vi "ActiveObject_QueueQueue_Process.vi"(0 "reference in":refnum<class>, 5 "error in (no error)":errorcluster) -> (14 "reference out":refnum<class>, 19 "error out":errorcluster)   [LabVIEW 2010]
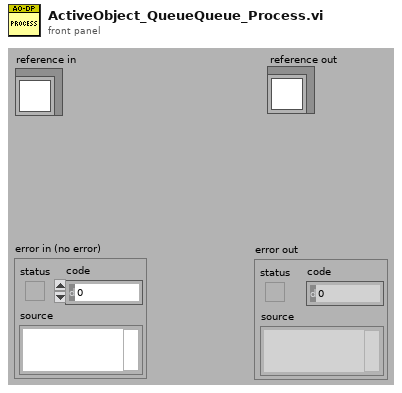
[diagram p1: front panel]
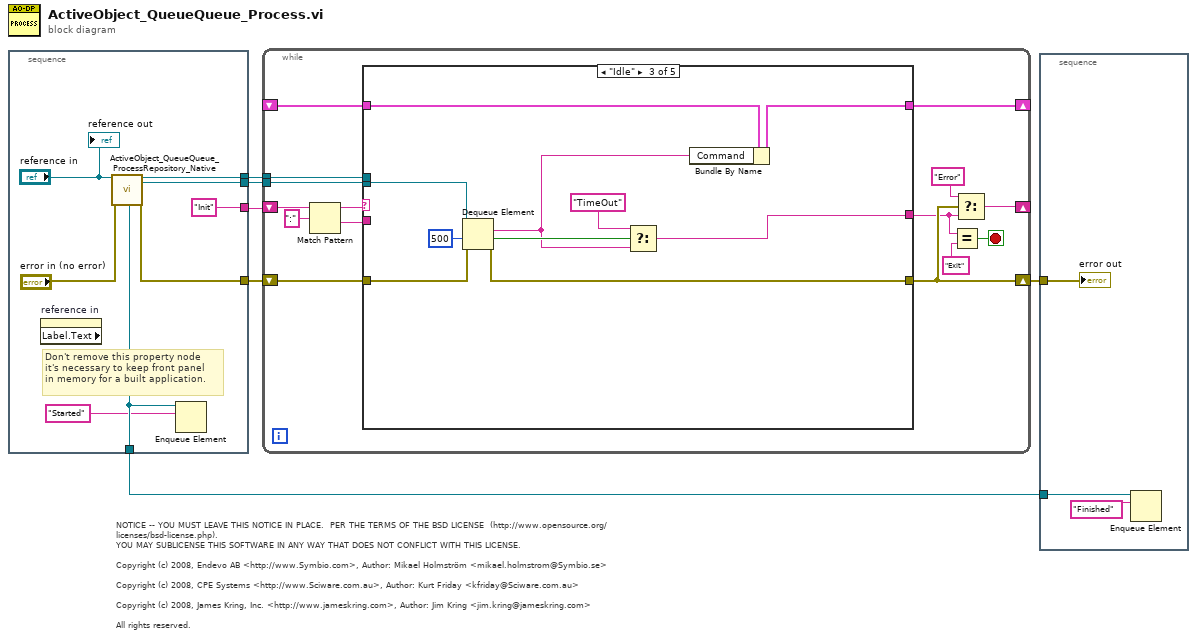
[diagram p0: block diagram]
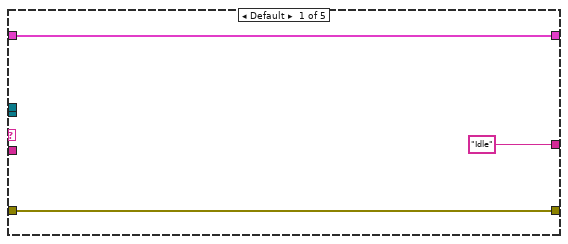
[diagram p2: hidden frame]
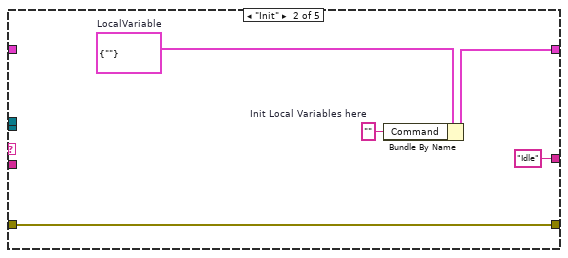
[diagram p3: hidden frame]
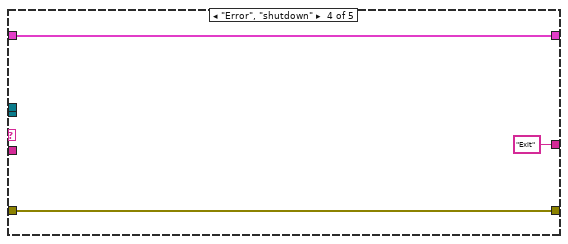
[diagram p4: hidden frame]
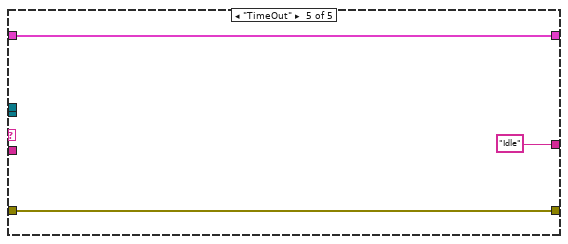
[diagram p5: hidden frame]
diagram:
  # "NOTICE -- YOU MUST LEAVE THIS NOTICE IN PLACE.  PER THE TERMS OF THE BSD LICENSE  (http://www.opensource.org/licenses/bsd-license.php).\nYOU MAY SUBLICENSE THIS SOFTWARE IN ANY WAY THAT DOES NOT CONFLICT WITH THIS LICENSE.\n\nCopyright (c) 2008, Endevo AB <http://www.Symbio.com>, Author: Mikael Holmström <mikael.holmstrom@Symbio.se>\n\nCopyright (c) 2008, CPE Systems <http://www.Sciware.com.au>, Author: Kurt Friday <kfriday@Sciware.com.au>\n\nCopyright (c) 2008, James Kring, Inc. <http://www.jameskring.com>, Author: Jim Kring <jim.kring@jameskring.com>\n\nAll rights reserved."
  n1 = stacked-sequence {
    tunnel: [w11] -> w6
    tunnel: [w14] -> w4
    tunnel: [w10] -> w3
    tunnel: [w8] -> w2
    tunnel: ["Init"] -> w1
    frame #0 {
      # "Don't remove this property node\nit's necessary to keep front panel\nin memory for a built application."
      n2 = property on="reference in" class="LVClassControl (strict)" props=["Label", "Text"]() -> ()  [unwired: 2 in, 3 out]
      n3 = call "ActiveObject_QueueQueue_ProcessRepository_Native.vi"("reference in"="reference in", "error in (no error)"="error in (no error)") -> ("ProcessSyncQueue"=w8:refnum<queue>, "reference out"=w14:refnum<class>, "ToProcessQueue"=w10:refnum<queue>, "error out"=w11:errorcluster)  [unwired: 11 in, 3 out]
      n4 = Enqueue Element(queue=w8, element="Started") -> ()  [unwired: 2 in, 3 out]
      "reference out" <- "reference in"
    }
  }
  n5 = while {
    shift-right: [w22] -> w5
    shift-left: w6 -> [w27]
    tunnel: w4 -> [w28]
    tunnel: w3 -> [w29]
    shift-right: [w20] -> _
    shift-left: w1 -> [w25]
    shift-right: [w16] -> _
    shift-left: _ -> [w15]
    stop <- w17 stop-if-true
    n6 = Match Pattern(string=w25, regular expression=":") -> (before substring=w24:string, after substring=w23:string)  [unwired: 1 in, 2 out]
    n7 = case shown="\"Idle\"" w24 {
      tunnel: w27 -> [w32 w34 w45 w50 w53]
      tunnel: [w32 w34 w44 w50 w53] -> w22
      tunnel: w29 -> [_ _ w46 _ _]
      tunnel: w28 -> [_ _ _ _ _]
      tunnel: w23 -> [_ _ _ _ _]
      tunnel: ["Idle" ("t") "Idle" ("t") w41 "Exit" ("y") "Idle" ("t")] -> w19
      tunnel: [w30 w36 w38 w48 w51] -> w16
      tunnel: w15 -> [w30 _ w39 w48 w51]
      frame Default {
      }
      frame "Init" {
        w35 = ""  # Init Local Variables here
        w37 = cluster{"Command":string} {"Command"=""}  # LocalVariable
        n8 = Bundle By Name(cluster=w37, "Command"=w35) -> (w36:cluster{"Command":string})
      }
      frame "Idle" {
        n9 = Dequeue Element(queue=w46, timeout in ms (-1)=500, error in (no error)=w45) -> (element=w40:string, timed out?=w43:bool, error out=w44:errorcluster)  [unwired: 1 out]
        n10 = Select(t="TimeOut", s=w43, f=w40) -> (s? t:f=w41:string)
        n11 = Bundle By Name(cluster=w39, "Command"=w40) -> (w38:cluster{"Command":string})
      }
      frame "Error", "shutdown" {
      }
      frame "TimeOut" {
      }
    }
    n12 = Equal?(x=w19, y="Exit") -> (x = y?=w17:bool)
    n13 = Select(t="Error", s=w22, f=w19) -> (s? t:f=w20:string)
  }
  n14 = stacked-sequence {
    tunnel: w5 -> [w56]
    tunnel: w2 -> [w55]
    frame #0 {
      n15 = Enqueue Element(queue=w55, element="Finished") -> ()  [unwired: 2 in, 3 out]
      "error out" <- w56
    }
  }
